vi "grabSetup.vi"(0 "HGF_IMAQDevice":refnum<class "HGF_IMAQDevice.lvclass">, 5 "error in (no error)":errorcluster, 6 "Region of Interest":i32[](array[numeric]), 7 "Step x":i32=-1, 8 "Channel":i32=-1, 9 "Step y":i32=-1) -> (14 "dup HGF_IMAQDevice":refnum<class "HGF_IMAQDevice.lvclass">, 19 "error out":errorcluster)   [LabVIEW 2014, in "HGF_IMAQ.lvlib" / "HGF_IMAQDevice.lvclass"]
doc: "Starts a grab acquisition. This VI performs a continuous acquisition that provides access to the most recently acquired image.\n\nParameter are used for framegrabber, only, and can be ignored for IMAQdx and IMAQ for USB."
uses:
  HGF_IMAQDevice.lvclass
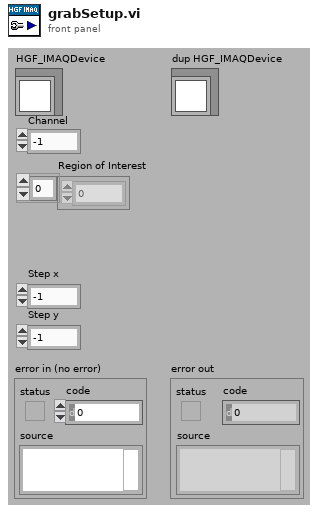
[diagram p1: front panel]
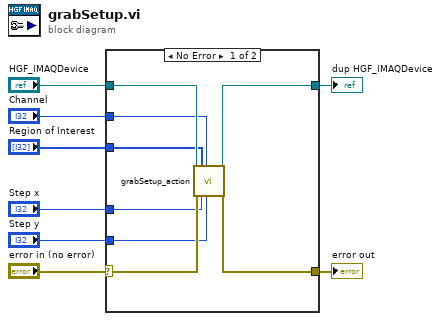
[diagram p0: block diagram]
diagram:
  n1 = case shown="No Error" "error in (no error)" {
    selector: "error in (no error)" -> [w16 w18]
    tunnel: [w15 w18] -> w7
    tunnel: [w13 w17] -> w5
    tunnel: "HGF_IMAQDevice" -> [w14 w17]
    tunnel: "Channel" -> [w12 _]
    tunnel: "Region of Interest" -> [w11 _]
    tunnel: "Step x" -> [w10 _]
    tunnel: "Step y" -> [w9 _]
    frame No Error {
      n2 = call-dynamic "grabSetup_action.vi"("HGF_IMAQDevice"=w14, "error in (no error)"=w16, "Region of Interest"=w11, "Step x"=w10, "Channel"=w12, "Step y"=w9) -> ("dup HGF_IMAQDevice"=w13:refnum<class "HGF_IMAQDevice.lvclass">, "error out"=w15:errorcluster)  [unwired: 12 in]
    }
    frame Error {
    }
  }
  "error out" <- w7
  "dup HGF_IMAQDevice" <- w5
